vi "User.vi"() -> ()   [LabVIEW 2023]
uses:
  Tab_typeDef_user.ctl
  Global 1.vi
  <vilib>/Utility/file.llb/Read Delimited Spreadsheet (string).vi
  <vilib>/Utility/file.llb/Write Delimited Spreadsheet (string).vi
panel:
  in  "Tab Control":T1(tab)=enum."Registration"
  out "String":string
  in  "register_btn":bool
  in  "login_btn":bool
  in  "password_login":string
  in  "username_login":string
  in  "home_btn":bool
  in  "Location_of_locker":u16(ring) items=["Choose location", "ul. Arkuszowa 109, 01-934 Warszawa", "ul. Polczynska 104, 01-302 Warszawa"]
  in  "Send_Button":bool
  in  "Receive_Button":bool caption="Send_Button"
  in  "back_to_login_btn":bool
  out "rgstr_status":string
  in  "email_address_rgstr":string
  in  "last_name_rgstr":string
  in  "first_name_rgstr":string
  in  "register_btn_rgstr":bool
  in  "password_rgstr":string
  in  "username_rgstr":string
  in  "pickup_btn_rcv":bool
  in  "menu_btn_rcv":bool
  in  "pickup_code_rcv_1":string
  in  "phone_receiver_rcv_1":string
  in  "radio_btn_sizes_of_parcel 2":T2(radio)
  in  "Location_of_locker_rcp":u16(ring) items=["Choose location", "ul. Arkuszowa 109, 01-934 Warszawa", "ul. Polczynska 104, 01-302 Warszawa"]
  in  "Location_of_locker_sender_send":u16(ring) items=["Choose location", "ul. Arkuszowa 109, 01-934 Warszawa", "ul. Polczynska 104, 01-302 Warszawa"]
  in  "recipient_phone_send":string
  in  "sender_phone_number_send":string
  in  "next_btn_send":bool
  in  "back_btn_send":bool
  # "User:"
  # "Login"
  # "Thanks for choosing\nParcelFast"
  # "Username:"
  # "Use our system in two steps:"
  # "Password:"
  # "1. Select your current location: B"
  # "2. Do you want to send or receive a package?"
  # "or Register"
  # "Registration"
  # "First Name:"
  # "Last Name:"
  # "Email Address:"
  # "Username:"
  # "Password:"
  # "Fill in the required gaps below:"
  # "Phone number:"
  # "Pickup-code:"
  # "Confirm your details:"
  # "You:"
  # "Phone number:"
  # "Destination:"
  # "Recipient:"
  # "Phone number:"
  # "Destination:"
  # "Min size"
  # "Medium size"
  # "Big size"
  # "Price 15,00 zl"
  # "Price 18,99 zl"
  # "Price 18,99 zl"
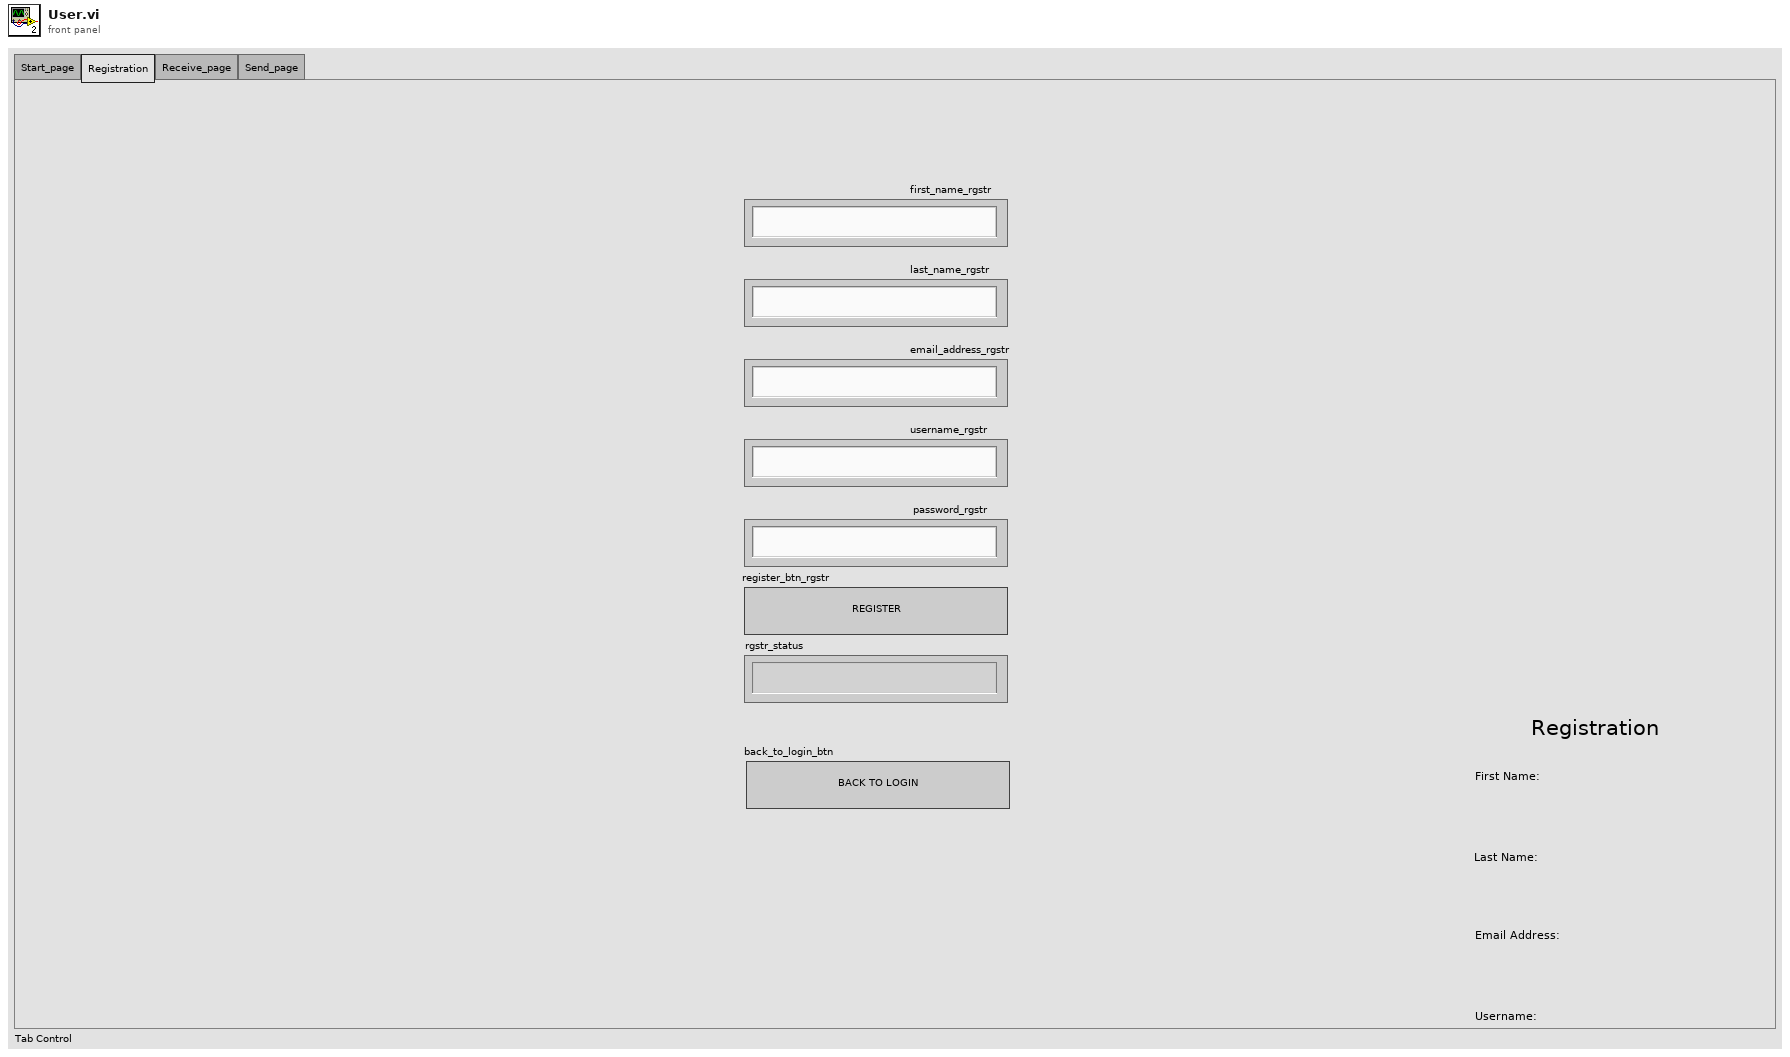
[diagram p1: front panel]
types:
  T1 = enum32{"Start_page", "Registration", "Receive_page", "Send_page"}
  T2 = enum32{"Radio Selection 1", "Radio Selection 2", "Radio Selection 3"}
  T3 = typedef "Tab_typeDef_user.ctl" = enum32{"Start_page", "Registration", "Receive_page", "Send_page"}
  T4 = cluster{bool, "tab_control_user ":T3, "phone_receiver":string, "pickup_code_receiver":string, "time_start_rcv":timestamp, "time_end_rcv":timestamp, "time_start_send":timestamp, "time_end_send":timestamp, "your_phone_receiver":string, "recipients_phone_receiver":string, "radio_btn_size":i32, "Probe":i32}
  T5 = enum16{"open", "replace", "create", "open or create", "replace or create", "replace or create with confirmation"}
  T6 = typedef "Tab_typeDef_lock_state.ctl" = u16
  T7 = cluster{"id_locker":i32, "lock_state":T6, "array_of_boxes_of_locker":cluster{"parcel_end_time":timestamp, "parcel_placement_time":timestamp, "box_filling":dbl, "adres_to send_parcel":i32}[][], "num_parcel":dbl[]}[]
  T8 = cluster{"id_locker":i32, "lock_state":T6, "array_of_boxes_of_locker":cluster{"parcel_end_time":timestamp, "parcel_placement_time":timestamp, "box_filling":dbl, "adres_to send_parcel":i32}[][], "num_parcel":dbl[]}
  T9 = cluster{"parcel_end_time":timestamp, "parcel_placement_time":timestamp, "box_filling":dbl, "adres_to send_parcel":i32}[][]
  T10 = cluster{"parcel_end_time":timestamp, "parcel_placement_time":timestamp, "box_filling":dbl, "adres_to send_parcel":i32}[]
  T11 = cluster{"parcel_end_time":timestamp, "parcel_placement_time":timestamp, "box_filling":dbl, "adres_to send_parcel":i32}
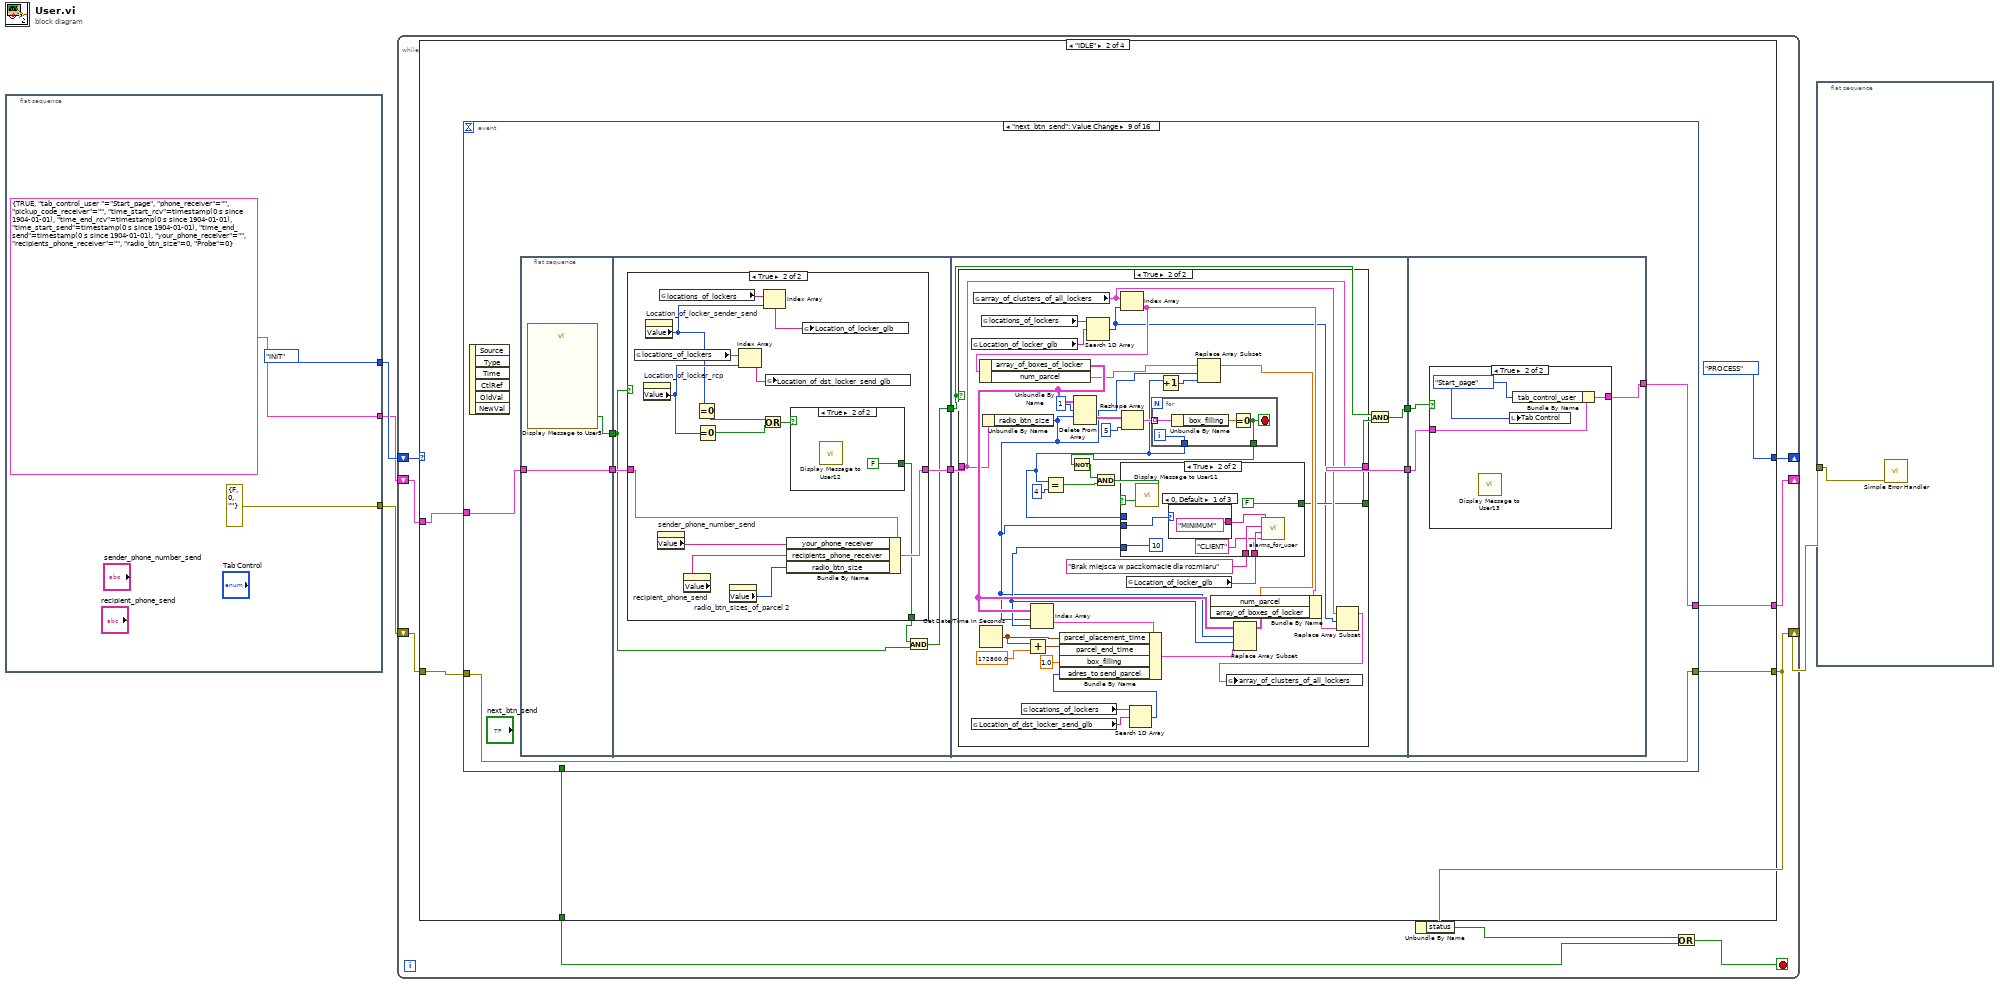
[diagram p0: block diagram]
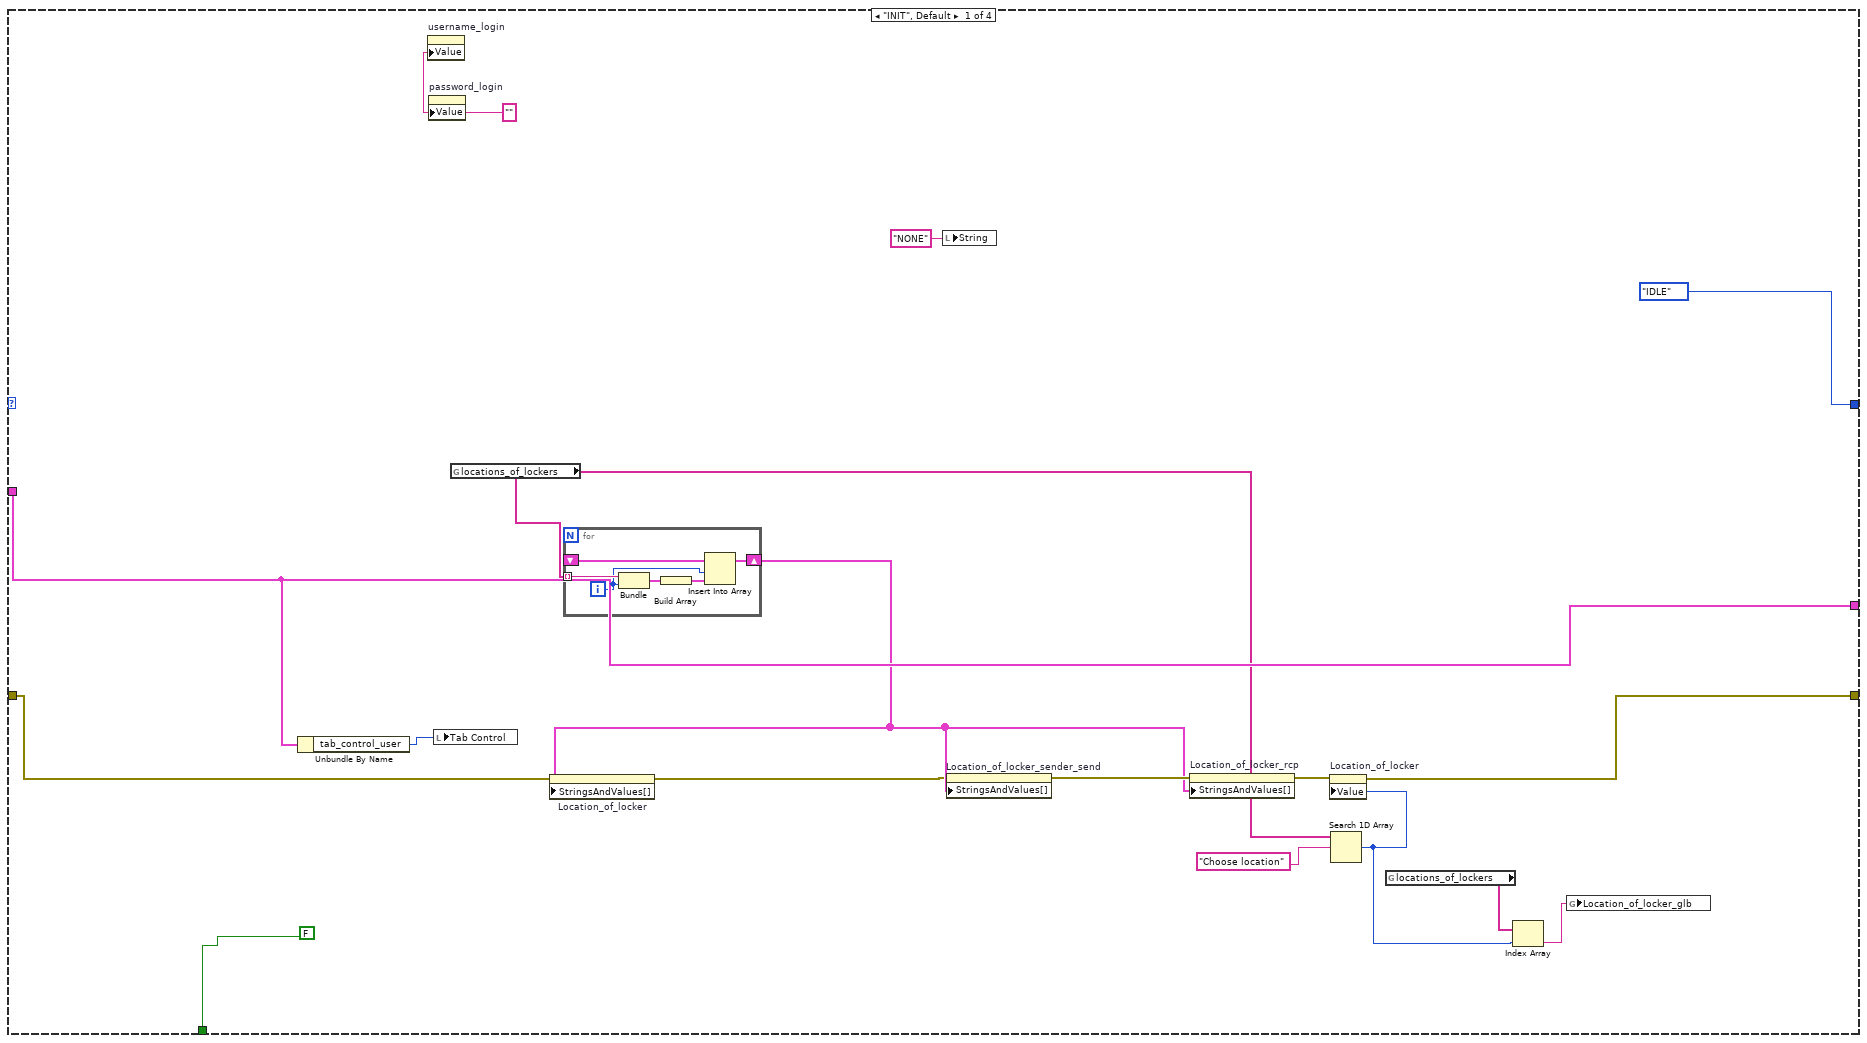
[diagram p2: hidden frame]
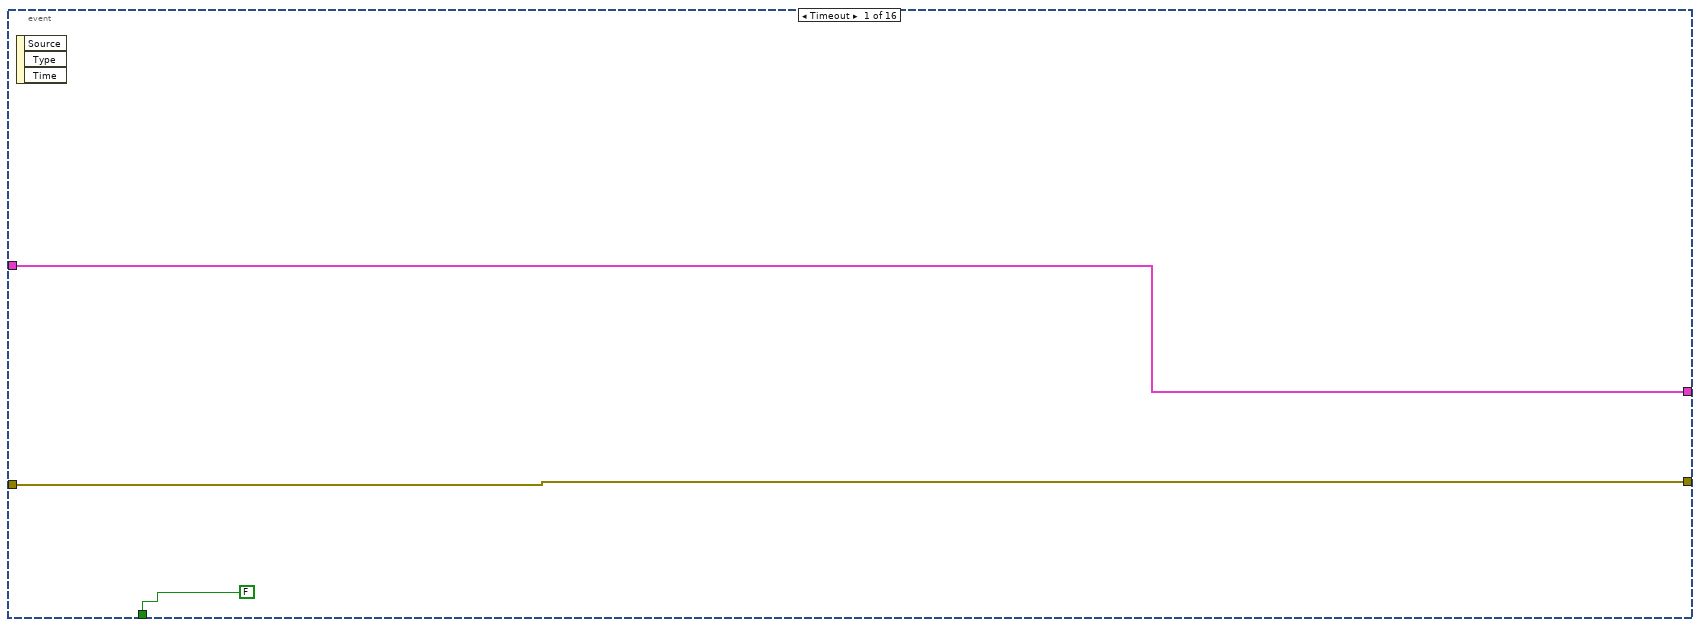
[diagram p3: hidden frame]
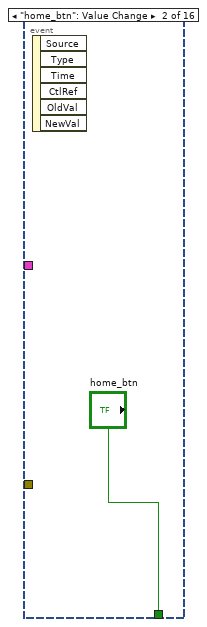
[diagram p4: hidden frame]
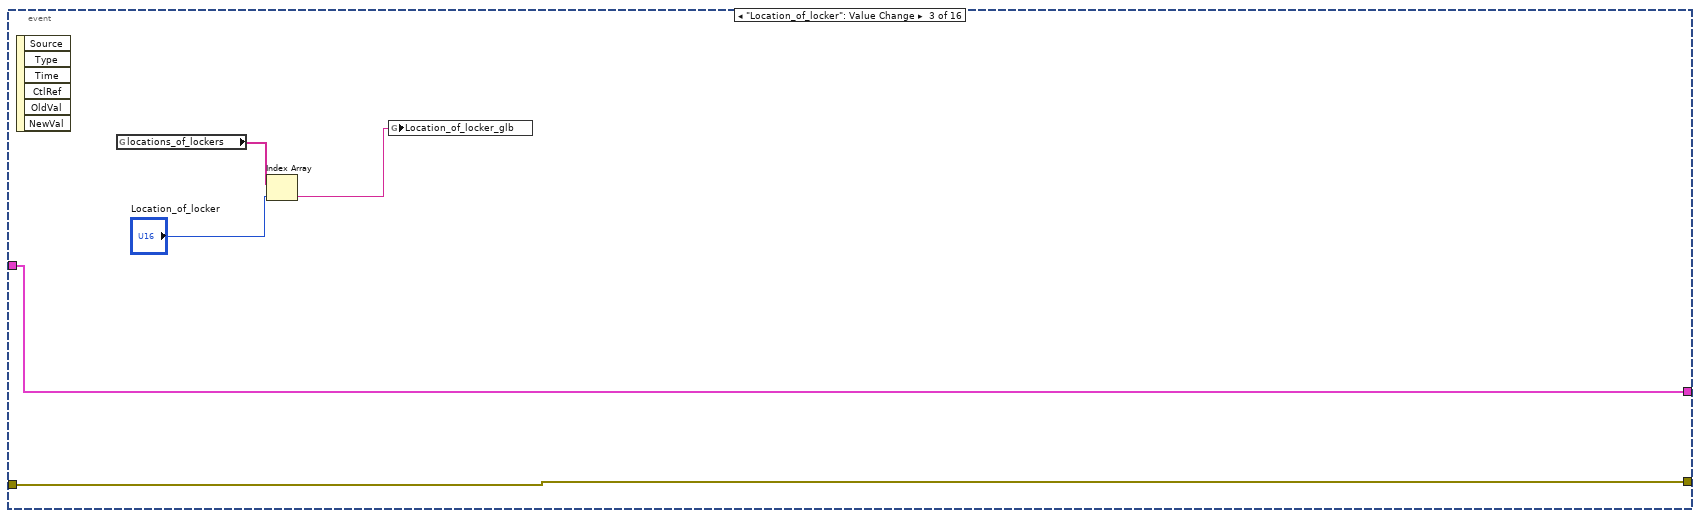
[diagram p5: hidden frame]
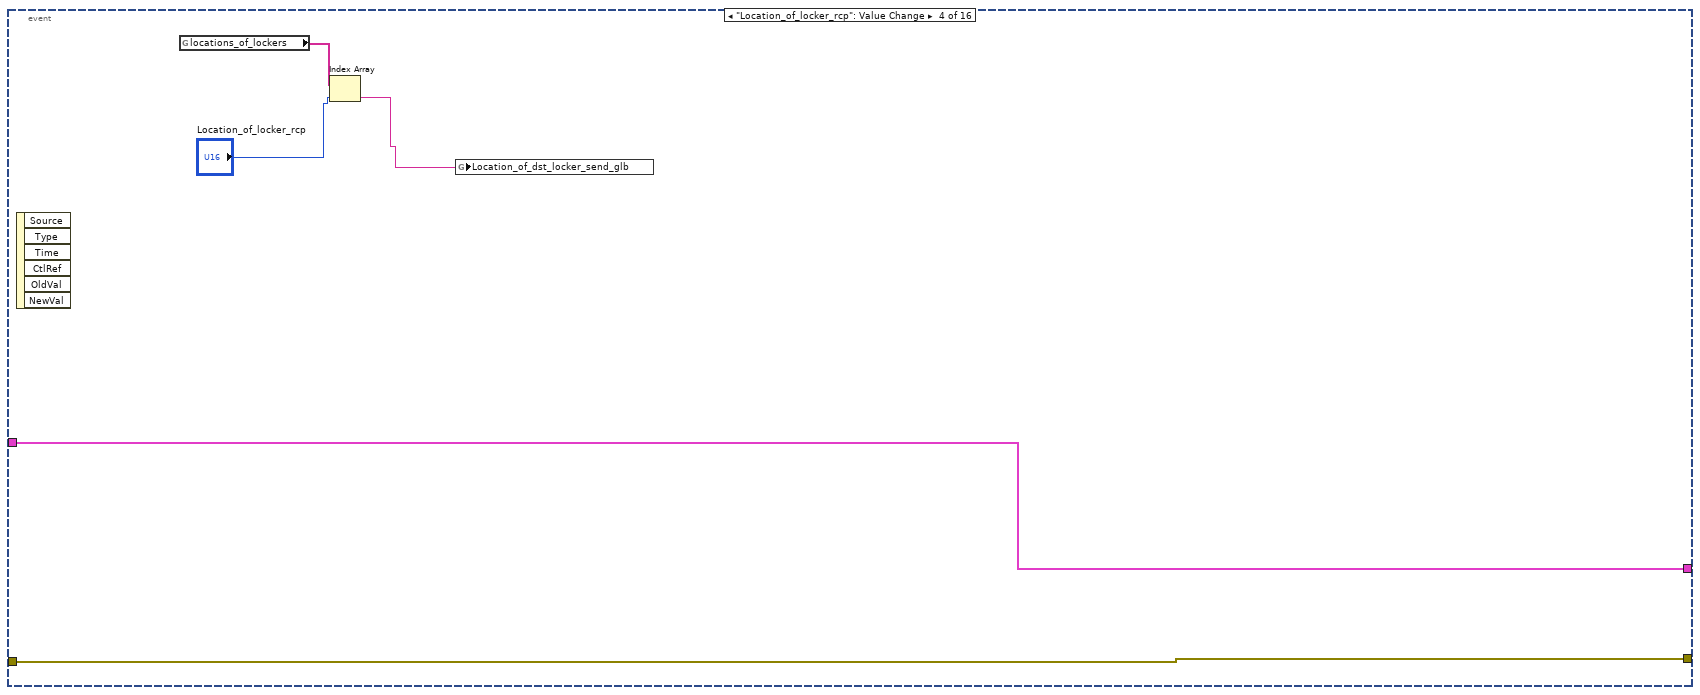
[diagram p6: hidden frame]
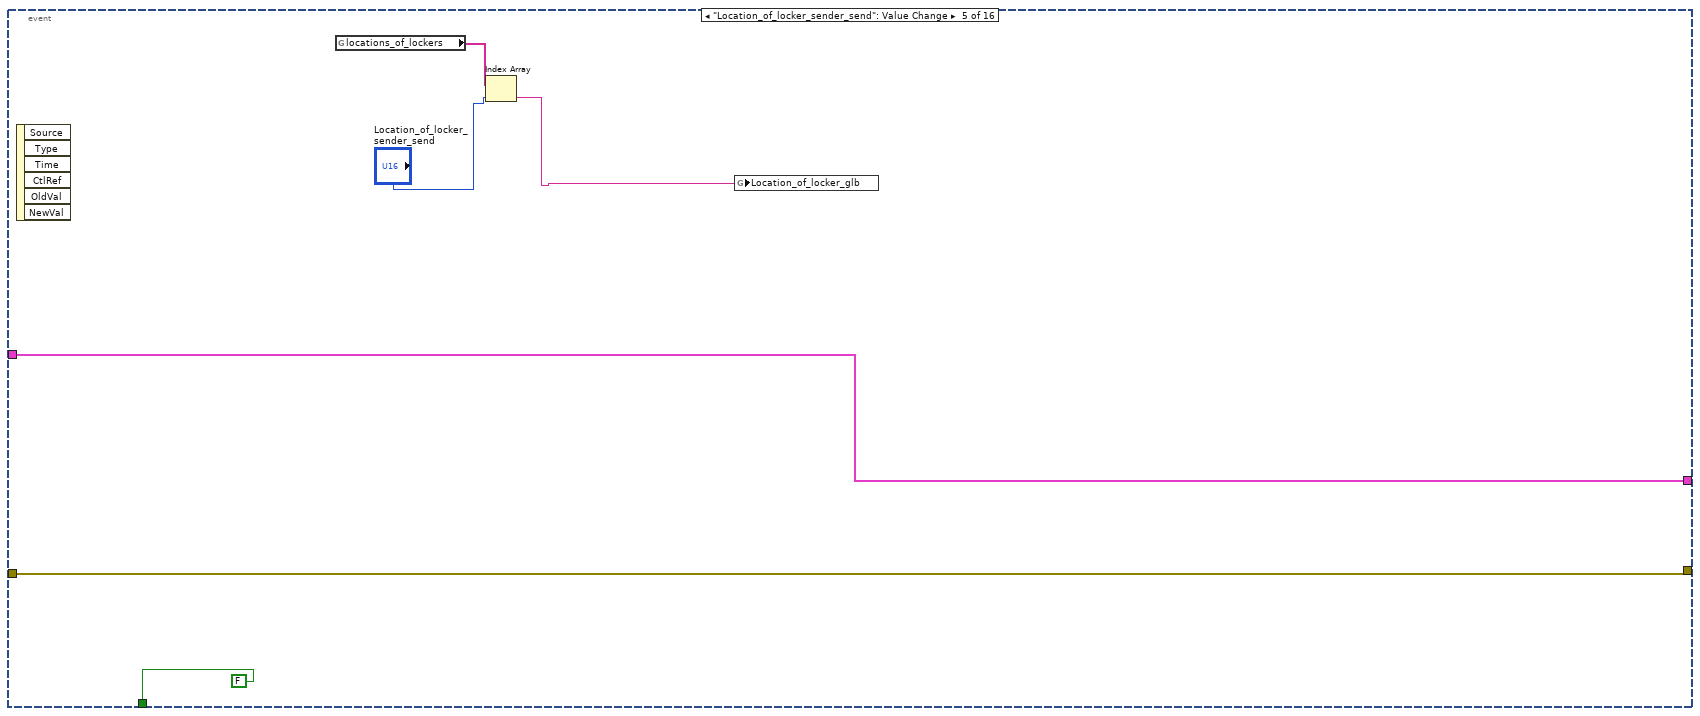
[diagram p7: hidden frame]
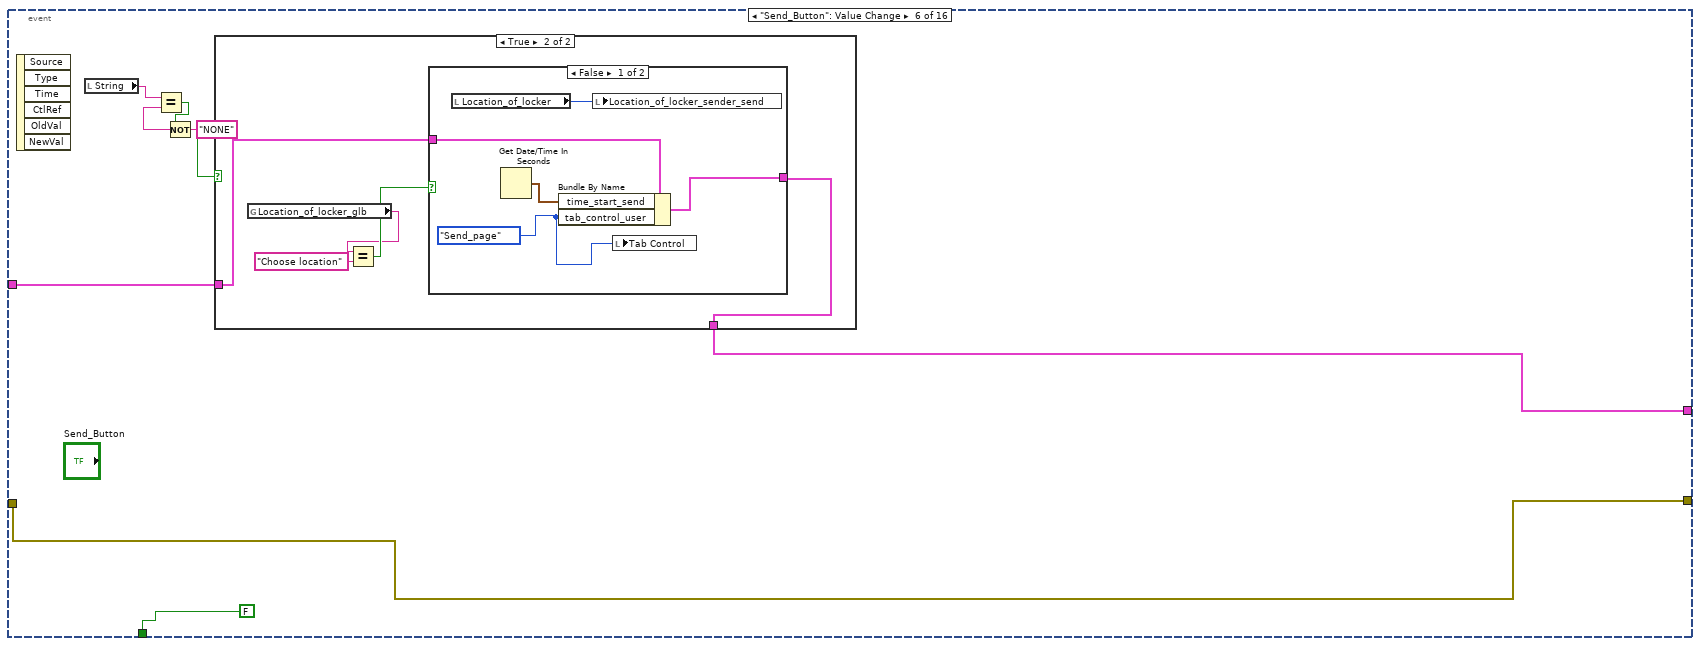
[diagram p8: hidden frame]
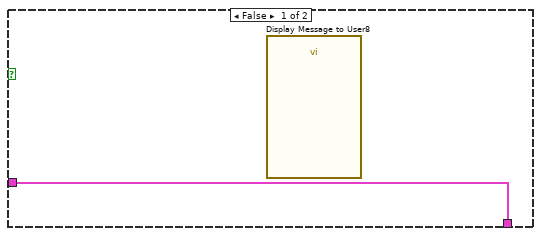
[diagram p9: hidden frame]
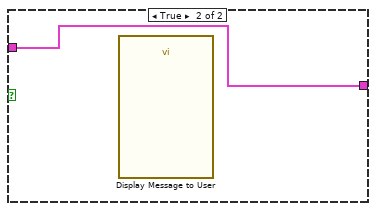
[diagram p10: hidden frame]
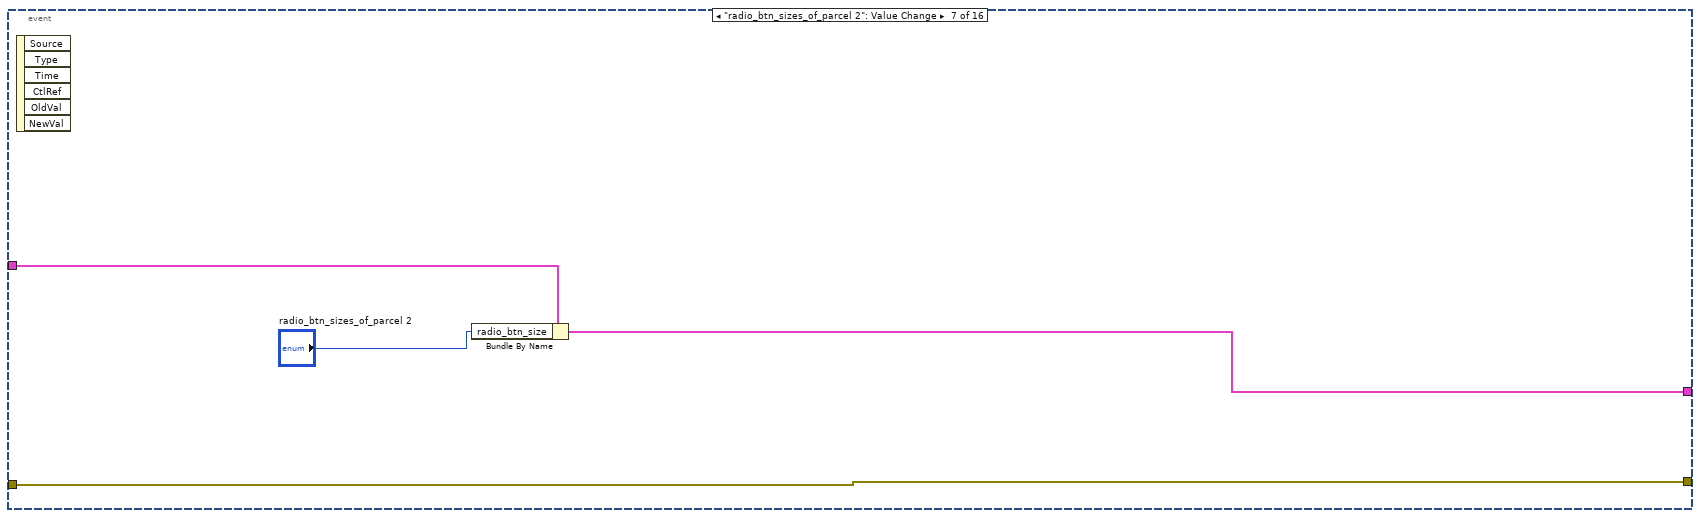
[diagram p11: hidden frame]
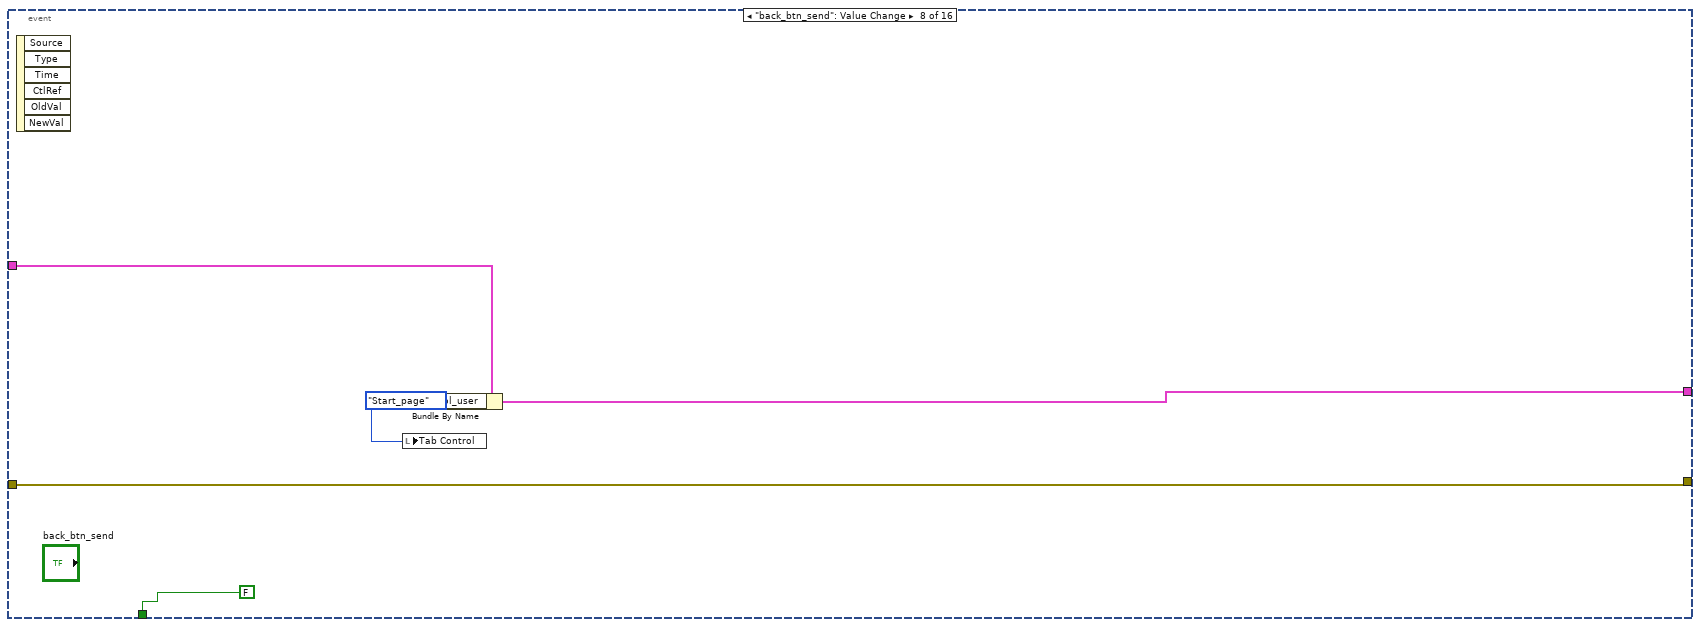
[diagram p12: hidden frame]
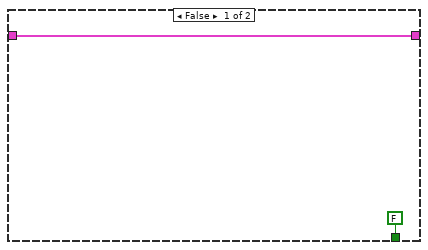
[diagram p13: hidden frame]
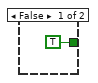
[diagram p14: hidden frame]
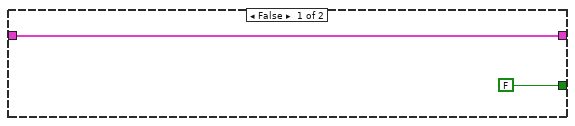
[diagram p15: hidden frame]
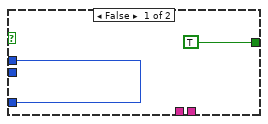
[diagram p16: hidden frame]
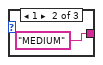
[diagram p17: hidden frame]
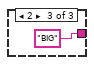
[diagram p18: hidden frame]
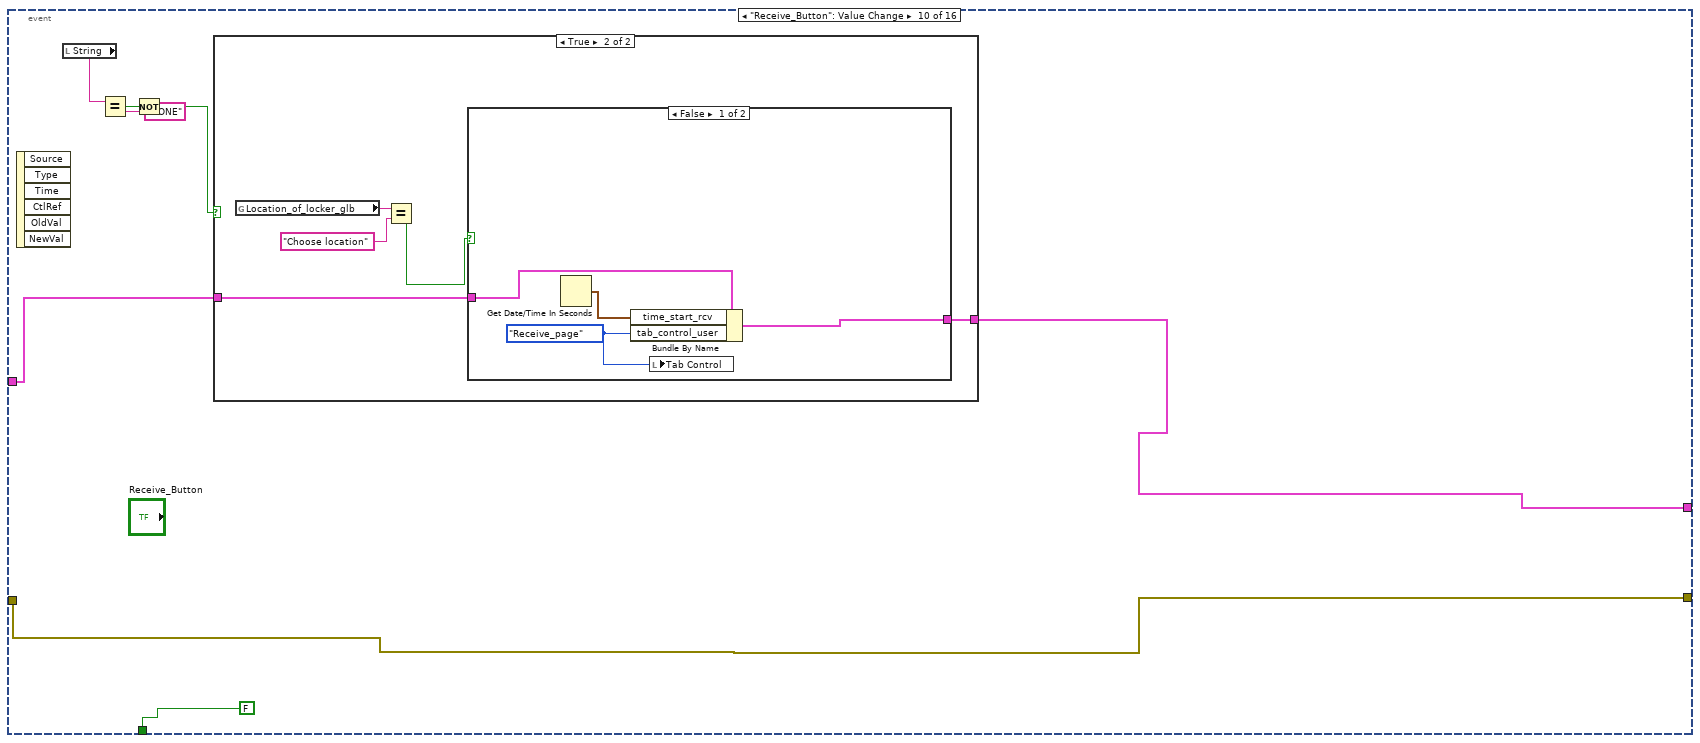
[diagram p20: hidden frame]
diagram:
  n1 = flat-sequence {
    tunnel: [errorcluster {"status"=FALSE, "code"=0, "source"=""} ("error constant")] -> w3
    tunnel: [enum16{"INIT", "IDLE", "PROCESS", "EXIT"}."INIT"] -> w4
    tunnel: [T4 {TRUE, "tab_control_user "=enum."Start_page", "phone_receiver"="", "pickup_code_receiver"="", "time_start_rcv"=timestamp(0 s since 1904-01-01), "time_end_rcv"=timestamp(0 s since 1904-01-01), "time_start_send"=timestamp(0 s since 1904-01-01), "time_end_send"=timestamp(0 s since 1904-01-01), "your_phone_receiver"="", "recipients_phone_receiver"="", "radio_btn_size"=0, "Probe"=0}] -> w1
    frame #0 {
    }
  }
  n2 = while {
    shift-right: [w15] -> _
    shift-left: w4 -> [w16]
    shift-right: [w14] -> _
    shift-left: w1 -> [w9]
    shift-right: [w11] -> w2
    shift-left: w3 -> [w8]
    stop <- w10 stop-if-true
    n3 = case shown="\"IDLE\"" w16 {
      tunnel: [enum16{"INIT", "IDLE", "PROCESS", "EXIT"}."IDLE" enum16{"INIT", "IDLE", "PROCESS", "EXIT"}."PROCESS" enum16{"INIT", "IDLE", "PROCESS", "EXIT"}."IDLE" enum16{"INIT", "IDLE", "PROCESS", "EXIT"}."EXIT"] -> w15
      tunnel: [FALSE ("stop") w44 FALSE ("stop") TRUE ("stop")] -> w12
      tunnel: [w31 w43 w395 w399] -> w14
      tunnel: [w21 w41 w394 w398] -> w11
      tunnel: w9 -> [w31 w42 w395 w399]
      tunnel: w8 -> [w29 w40 w394 w398]
      frame "INIT", Default {
        w17 = "" ("password_login")
        n4 = Unbundle By Name(w31) -> ("tab_control_user"=w30:T3)
        n5 = property on="username_login" class="Str"("Value"=w17) -> ()  [unwired: 2 in, 2 out]
        n6 = property on="password_login" class="Str"("Value"=w17) -> ()  [unwired: 2 in, 2 out]
        n7 = local write "Tab Control"(w30) -> ()
        n8 = global read "Global 1.vi" "locations_of_lockers"() -> (w23:string[])
        n9 = for {
          tunnel: w23 -> [w39] mode=indexing
          shift-right: [w36] -> w25
          shift-left: _ -> [w37]
          i -> [w34]
          n10 = Bundle("String"=w39, w34) -> (w38:cluster{"String":string, i32})  [unwired: 1 in]
          n11 = Build Array(w38) -> (w35:cluster{"String":string, i32}[])
          n12 = Insert Into Array(array=w37, index=w34, new element=w35) -> (w36:cluster{"String":string, i32}[])
        }
        n13 = property on="Location_of_locker" class="Ring (strict)"(error in=w29, "StringsAndValues[]"=w25) -> (error out=w22:errorcluster)  [unwired: 1 in, 1 out]
        n14 = local write "String"("NONE" ("String")) -> ()
        n15 = property on="Location_of_locker_sender_send" class="Ring (strict)"(error in=w22, "StringsAndValues[]"=w25) -> (error out=w27:errorcluster)  [unwired: 1 in, 1 out]
        n16 = property on="Location_of_locker_rcp" class="Ring (strict)"(error in=w27, "StringsAndValues[]"=w25) -> (error out=w26:errorcluster)  [unwired: 1 in, 1 out]
        n17 = Search 1D Array(1D array=w23, element="Choose location" ("new element/subarray")) -> (index of element=w18:i32)  [unwired: 1 in]
        n18 = property on="Location_of_locker" class="Ring (strict)"(error in=w26, "Value"=w18) -> (error out=w21:errorcluster)  [unwired: 1 in, 1 out]
        n19 = global read "Global 1.vi" "locations_of_lockers"() -> (w20:string[])
        n20 = Index Array(array=w20, index=w18) -> (element=w19:string)
        n21 = global write "Global 1.vi" "Location_of_locker_glb"(w19) -> ()
      }
      frame "IDLE" {
        n22 = event shown="[8] \"next_btn_send\": Value Change" {
          selector: _ -> [_ _ _ _ _ _ _ _ _ _ _ _ _ _ _ _]
          dyn-events: _ -> [_ _ _ _ _ _ _ _ _ _ _ _ _ _ _ _]
          timeout: _ -> [_ _ _ _ _ _ _ _ _ _ _ _ _ _ _ _]
          tunnel: [FALSE ("stop") "home_btn" _ _ FALSE ("home_btn") FALSE ("home_btn") _ FALSE ("home_btn") _ FALSE ("home_btn") FALSE ("home_btn") _ _ _ _ _] -> w44
          tunnel: [w47 _ w54 w58 w63 w71 w87 w91 w99 w203 w217 w225 w228 w306 _ w391] -> w43
          tunnel: w42 -> [w47 _ w54 w58 w63 w72 w89 w92 w102 w204 w218 w223 w231 w308 _ w393]
          tunnel: [w46 _ w53 w59 w64 w70 w86 w93 w103 w202 _ _ w226 w299 _ w388] -> w41
          tunnel: w40 -> [w46 _ w53 w59 w64 w70 w86 w93 w103 w202 _ _ w226 w300 _ w390]
          event Timeout {
            n23 = event-data() -> ()  [unwired: 1 in, 3 out]
          }
          event "home_btn": Value Change {
            n24 = event-data() -> ()  [unwired: 1 in, 6 out]
          }
          event "Location_of_locker": Value Change {
            n25 = event-data() -> ()  [unwired: 1 in, 6 out]
            n26 = global read "Global 1.vi" "locations_of_lockers"() -> (w51:string[])
            n27 = Index Array(array=w51, index="Location_of_locker") -> (element=w50:string)
            n28 = global write "Global 1.vi" "Location_of_locker_glb"(w50) -> ()
          }
          event "Location_of_locker_rcp": Value Change {
            n29 = event-data() -> ()  [unwired: 1 in, 6 out]
            n30 = global read "Global 1.vi" "locations_of_lockers"() -> (w57:string[])
            n31 = Index Array(array=w57, index="Location_of_locker_rcp") -> (element=w55:string)
            n32 = global write "Global 1.vi" "Location_of_dst_locker_send_glb"(w55) -> ()
          }
          event "Location_of_locker_sender_send": Value Change {
            n33 = event-data() -> ()  [unwired: 1 in, 6 out]
            n34 = global read "Global 1.vi" "locations_of_lockers"() -> (w62:string[])
            n35 = Index Array(array=w62, index="Location_of_locker_sender_send") -> (element=w60:string)
            n36 = global write "Global 1.vi" "Location_of_locker_glb"(w60) -> ()
          }
          event "Send_Button": Value Change {
            n37 = event-data() -> ()  [unwired: 1 in, 6 out]
            n38 = local read "String"() -> (w69:string)
            n39 = Equal?(x=w69, y="NONE") -> (x = y?=w67:bool)
            n40 = Not(x=w67) -> (.not. x?=w66:bool)
            n41 = case shown="True" w66 {
              tunnel: w72 -> [w74 w77]
              tunnel: [w74 w76] -> w71
              frame False {
                n42 = call "Display Message to User8"() -> ()  [unwired: 10 in, 2 out]
              }
              frame True {
                n43 = global read "Global 1.vi" "Location_of_locker_glb"() -> (w75:string)
                n44 = Equal?(x=w75, y="Choose location") -> (x = y?=w78:bool)
                n45 = case shown="False" w78 {
                  tunnel: w77 -> [w84 w85]
                  tunnel: [w83 w85] -> w76
                  frame False {
                    w81 = Tab_typeDef_user."Send_page" ("tab_control_user")
                    n46 = local read "Location_of_locker"() -> (w80:u16)
                    n47 = Get Date/Time In Seconds() -> (seconds since 1Jan1904=w82:timestamp)
                    n48 = Bundle By Name(cluster=w84, "time_start_send"=w82, "tab_control_user"=w81) -> (w83:T4)
                    n49 = local write "Location_of_locker_sender_send"(w80) -> ()
                    n50 = local write "Tab Control"(w81) -> ()
                  }
                  frame True {
                    n51 = call "Display Message to User"() -> ()  [unwired: 10 in, 2 out]
                  }
                }
              }
            }
          }
          event "radio_btn_sizes_of_parcel 2": Value Change {
            n52 = event-data() -> ()  [unwired: 1 in, 6 out]
            n53 = Bundle By Name(cluster=w89, "radio_btn_size"="radio_btn_sizes_of_parcel 2") -> (w87:T4)
          }
          event "back_btn_send": Value Change {
            w90 = Tab_typeDef_user."Start_page" ("tab_control_user")
            n54 = event-data() -> ()  [unwired: 1 in, 6 out]
            n55 = Bundle By Name(cluster=w92, "tab_control_user"=w90) -> (w91:T4)
            n56 = local write "Tab Control"(w90) -> ()
          }
          event "next_btn_send": Value Change {
            n57 = event-data() -> ()  [unwired: 1 in, 6 out]
            n58 = flat-sequence {
              tunnel: w102 -> [w105]
              tunnel: [w105] -> w101
              tunnel: [w104] -> w100
              tunnel: w101 -> [w110]
              tunnel: [w109] -> w98
              tunnel: [w106] -> w96
              tunnel: w100 -> [w107]
              tunnel: w98 -> [w134]
              tunnel: [w133] -> w97
              tunnel: w96 -> [w132]
              tunnel: [w131] -> w95
              tunnel: [w191] -> w99
              tunnel: w97 -> [w192]
              tunnel: w95 -> [w190]
              frame #0 {
                n59 = call "Display Message to User5"() -> ("OK"=w104:bool)  [unwired: 10 in, 1 out]
              }
              frame #1 {
                n60 = case shown="True" w107 {
                  tunnel: w110 -> [w112 w127]
                  tunnel: [w112 w124] -> w109
                  tunnel: [FALSE w113] -> w108
                  frame False {
                  }
                  frame True {
                    n61 = global read "Global 1.vi" "locations_of_lockers"() -> (w121:string[])
                    n62 = property on="Location_of_locker_rcp" class="Ring (strict)"() -> ("Value"=w118:u16)  [unwired: 2 in, 2 out]
                    n63 = property on="Location_of_locker_sender_send" class="Ring (strict)"() -> ("Value"=w116:u16)  [unwired: 2 in, 2 out]
                    n64 = property on="sender_phone_number_send" class="Str"() -> ("Value"=w126:string)  [unwired: 2 in, 2 out]
                    n65 = global read "Global 1.vi" "locations_of_lockers"() -> (w123:string[])
                    n66 = property on="recipient_phone_send" class="Str"() -> ("Value"=w125:string)  [unwired: 2 in, 2 out]
                    n67 = Equal To 0?(x=w116) -> (x = 0?=w115:bool)
                    n68 = Equal To 0?(x=w118) -> (x = 0?=w114:bool)
                    n69 = property on="radio_btn_sizes_of_parcel 2" class="RadioBtnsControl (strict)"() -> ("Value"=w119:T2)  [unwired: 2 in, 2 out]
                    n70 = Index Array(array=w121, index=w118) -> (element=w120:string)
                    n71 = Or(x=w115, y=w114) -> (x .or. y?=w117:bool)
                    n72 = Index Array(array=w123, index=w116) -> (element=w122:string)
                    n73 = global write "Global 1.vi" "Location_of_dst_locker_send_glb"(w120) -> ()
                    n74 = Bundle By Name(cluster=w127, "your_phone_receiver"=w126, "recipients_phone_receiver"=w125, "radio_btn_size"=w119) -> (w124:T4)
                    n75 = case shown="True" w117 {
                      tunnel: [TRUE FALSE] -> w113
                      frame False {
                      }
                      frame True {
                        n76 = call "Display Message to User12"() -> ()  [unwired: 10 in, 2 out]
                      }
                    }
                    n77 = global write "Global 1.vi" "Location_of_locker_glb"(w122) -> ()
                  }
                }
                n78 = And(x=w108, y=w107) -> (x .and. y?=w106:bool)
              }
              frame #2 {
                n79 = case shown="True" w132 {
                  tunnel: w134 -> [w136 w146]
                  tunnel: [w136 w146] -> w133
                  tunnel: [FALSE w147] -> w130
                  frame False {
                  }
                  frame True {
                    n80 = global read "Global 1.vi" "Location_of_locker_glb"() -> (w172:string)
                    n81 = global read "Global 1.vi" "Location_of_dst_locker_send_glb"() -> (w141:string)
                    n82 = global read "Global 1.vi" "array_of_clusters_of_all_lockers"() -> (w158:T7)
                    n83 = Get Date/Time In Seconds() -> (seconds since 1Jan1904=w164:timestamp)
                    n84 = global read "Global 1.vi" "locations_of_lockers"() -> (w173:string[])
                    n85 = Unbundle By Name(w146) -> ("radio_btn_size"=w139:i32)
                    n86 = global read "Global 1.vi" "locations_of_lockers"() -> (w142:string[])
                    n87 = Add(x=w164, y=172800.0) -> (x+y=w165:timestamp)
                    n88 = Search 1D Array(1D array=w173, element=w172) -> (index of element=w143:i32)  [unwired: 1 in]
                    n89 = Index Array(array=w158, index=w143) -> (element=w160:T8)
                    n90 = Unbundle By Name(w160) -> ("array_of_boxes_of_locker"=w162:T9, "num_parcel"=w155:dbl[])
                    n91 = Delete From Array(array=w162, length=1, index (row)=w139) -> (deleted portion=w170:T9)  [unwired: 1 in, 1 out]
                    n92 = Reshape Array(w170, 5 ("dimension size")) -> (w168:T10)
                    n93 = global read "Global 1.vi" "Location_of_locker_glb"() -> (w137:string)
                    n94 = Search 1D Array(1D array=w142, element=w141) -> (index of element=w140:i32)  [unwired: 1 in]
                    n95 = for {
                      tunnel: w168 -> [w189] mode=indexing
                      tunnel: [w187] -> w145
                      tunnel: [w186] -> w150
                      i -> [w187]
                      stop <- w186 stop-if-true
                      n96 = Unbundle By Name(w189) -> ("box_filling"=w188:dbl)
                      n97 = Equal To 0?(x=w188) -> (x = 0?=w186:bool)
                    }
                    n98 = Equal?(x=w145, y=4) -> (x = y?=w152:bool)
                    n99 = Not(x=w150) -> (.not. x?=w149:bool)
                    n100 = And(x=w149, y=w152) -> (x .and. y?=w151:bool)
                    n101 = case shown="True" w151 {
                      tunnel: w145 -> [w175 _]
                      tunnel: [w175 10] -> w148
                      tunnel: [TRUE FALSE] -> w147
                      tunnel: w139 -> [_ w180]
                      tunnel: "Brak miejsca w paczkomacie dla rozmiaru" -> [_ w178]
                      tunnel: w137 -> [_ w179]
                      frame False {
                      }
                      frame True {
                        n102 = call "Display Message to User11"() -> ()  [unwired: 10 in, 2 out]
                        n103 = case shown="0, Default" w180 {
                          tunnel: ["MINIMUM" "MEDIUM" "BIG"] -> w177
                          frame 0, Default {
                          }
                          frame 1 {
                          }
                          frame 2 {
                          }
                        }
                        n104 = call "alarms_for_user.vi"("name_user_option"="CLIENT", "adres"=w179, "texxt_alarm"=w178, "size_name"=w177) -> ()  [unwired: 8 in]
                      }
                    }
                    n105 = Index Array(array=w162, index (row)=w139, index (col)=w148) -> (element=w167:T11)
                    n106 = Bundle By Name(cluster=w167, "parcel_placement_time"=w164, "parcel_end_time"=w165, "box_filling"=1.0, "adres_to send_parcel"=w140) -> (w161:T11)
                    n107 = Increment(x=w145) -> (x+1=w144:i32)
                    n108 = Replace Array Subset(array=w155, new element=w144, index=w139) -> (w154:dbl[])
                    n109 = Replace Array Subset(array=w162, new element=w161, index (row)=w139, index (col)=w148) -> (w159:T9)
                    n110 = Bundle By Name(cluster=w160, "num_parcel"=w154, "array_of_boxes_of_locker"=w159) -> (w157:T8)
                    n111 = Replace Array Subset(array=w158, new element=w157, index=w143) -> (w156:T7)
                    n112 = global write "Global 1.vi" "array_of_clusters_of_all_lockers"(w156) -> ()
                  }
                }
                n113 = And(x=w132, y=w130) -> (x .and. y?=w131:bool)
              }
              frame #3 {
                n114 = case shown="True" w190 {
                  tunnel: w192 -> [w193 w196]
                  tunnel: [w193 w194] -> w191
                  frame False {
                  }
                  frame True {
                    w195 = Tab_typeDef_user."Start_page" ("tab_control_user")
                    n115 = call "Display Message to User13"() -> ()  [unwired: 10 in, 2 out]
                    n116 = local write "Tab Control"(w195) -> ()
                    n117 = Bundle By Name(cluster=w196, "tab_control_user"=w195) -> (w194:T4)
                  }
                }
              }
            }
          }
          event "Receive_Button": Value Change {
            n118 = event-data() -> ()  [unwired: 1 in, 6 out]
            n119 = local read "String"() -> (w200:string)
            n120 = Equal?(x=w200, y="NONE") -> (x = y?=w198:bool)
            n121 = Not(x=w198) -> (.not. x?=w197:bool)
            n122 = case shown="True" w197 {
              tunnel: w204 -> [w205 w207]
              tunnel: [w205 w206] -> w203
              frame False {
                n123 = call "Display Message to User9"() -> ()  [unwired: 10 in, 2 out]
              }
              frame True {
                n124 = global read "Global 1.vi" "Location_of_locker_glb"() -> (w209:string)
                n125 = Equal?(x=w209, y="Choose location") -> (x = y?=w208:bool)
                n126 = case shown="False" w208 {
                  tunnel: w207 -> [w214 w215]
                  tunnel: [w213 w215] -> w206
                  frame False {
                    w212 = Tab_typeDef_user."Receive_page" ("tab_control_user")
                    n127 = Get Date/Time In Seconds() -> (seconds since 1Jan1904=w211:timestamp)
                    n128 = Bundle By Name(cluster=w214, "time_start_rcv"=w211, "tab_control_user"=w212) -> (w213:T4)
                    n129 = local write "Tab Control"(w212) -> ()
                  }
                  frame True {
                    n130 = call "Display Message to User2"() -> ()  [unwired: 10 in, 2 out]
                  }
                }
              }
            }
          }
          event "menu_btn_rcv": Value Change {
            w216 = Tab_typeDef_user."Start_page" ("tab_control_user")
            n131 = event-data() -> ()  [unwired: 1 in, 6 out]
            n132 = Bundle By Name(cluster=w218, "tab_control_user"=w216) -> (w217:T4)
            n133 = local write "Tab Control"(w216) -> ()
          }
          event "pickup_btn_rcv": Value Change {
            w224 = Tab_typeDef_user."Start_page" ("tab_control_user")
            n134 = event-data() -> ()  [unwired: 1 in, 6 out]
            n135 = Bundle By Name(cluster=w223, "phone_receiver"="phone_receiver_rcv_1", "pickup_code_receiver"="pickup_code_rcv_1") -> (w220:T4)
            n136 = Bundle By Name(cluster=w220, "tab_control_user"=w224) -> (w225:T4)
            n137 = local write "Tab Control"(w224) -> ()
          }
          event "login_btn": Value Change {
            n138 = event-data() -> ()  [unwired: 1 in, 6 out]
            n139 = call <vilib>:"Application Directory.vi"() -> ("Application Directory"=w237:path)
            n140 = Path To String(path=w237) -> (string=w236:string)
            n141 = Concatenate Strings(w236, "\\databases\\") -> (w234:string)
            n142 = String To Path(string=w234) -> (path=w233:path)
            n143 = Build Path(base path=w233, name or relative path="Clients_database.csv") -> (appended path=w232:path)
            n144 = call-poly <vilib>:"Read Delimited Spreadsheet.vi"("file path (dialog if empty)"=w232, "delimiter (\\t)"="," ("delimiter (\\t)")) -> ("all rows"=w239:string[][])  [unwired: 8 in, 5 out]
            n145 = for {
              tunnel: w239 -> [w297] mode=indexing
              tunnel: "username_login" -> [w296]
              tunnel: "password_login" -> [w295]
              tunnel: [w292] -> w227
              stop <- w292 stop-if-true
              n146 = Index Array(array=w297) -> (element #4=w290:string, element #5=w291:string)  [unwired: 5 in, 3 out]
              n147 = Equal?(x=w290, y=w296) -> (x = y?=w294:bool)
              n148 = Equal?(x=w291, y=w295) -> (x = y?=w293:bool)
              n149 = And(x=w294, y=w293) -> (x .and. y?=w292:bool)
            }
            n150 = case shown="False" w227 {
              tunnel: w231 -> [w244 w289]
              tunnel: [w245 w288] -> w228
              tunnel: "username_login" -> [w252 w286]
              tunnel: "password_login" -> [w249 _]
              frame False {
                n151 = Unbundle By Name(w244) -> ("Probe"=w241:i32)
                n152 = Equal?(x=w241, y=3) -> (x = y?=w242:bool)
                n153 = case shown="True" w242 {
                  tunnel: [w255 w258] -> w245
                  tunnel: w244 -> [w256 w259]
                  tunnel: w241 -> [w253 _]
                  frame False {
                    n154 = Increment(x=w253) -> (x+1=w254:i32)
                    n155 = Bundle By Name(cluster=w256, "Probe"=w254) -> (w255:T4)
                  }
                  frame True {
                    n156 = Bundle By Name(cluster=w259, "Probe"=0) -> (w258:T4)
                    n157 = call <vilib>:"Application Directory.vi"() -> ("Application Directory"=w266:path)
                    n158 = Path To String(path=w266) -> (string=w265:string)
                    n159 = Concatenate Strings(w265, "\\alarms_events\\") -> (w263:string)
                    n160 = String To Path(string=w263) -> (path=w262:path)
                    n161 = Build Path(base path=w262, name or relative path="Alarms.txt") -> (appended path=w261:path)
                    n162 = Open/Create/Replace File(file path (use dialog)=w261, operation (0:open)=T5."open or create", access (0:read/write)=enum16{"read/write", "read-only", "write-only"}."write-only") -> (refnum out=w284:refnum<file>, error out=w285:errorcluster)  [unwired: 3 in, 1 out]
                    n163 = Get Date/Time String() -> (date string=w273:string, time string=w271:string)  [unwired: 3 in]
                    n164 = Set File Position(refnum=w284, from (0:start)=enum16{"start", "end", "current"}."end", error in=w285) -> (refnum out=w281:refnum<file>, error out=w280:errorcluster)  [unwired: 1 in]
                    n165 = Format Into String(format string="%s %s %s %s %s %s %s %s", "CLIENT" ("format string"), "Date:" ("format string"), w273, "Time:" ("format string"), w271, "ALARM: " ("format string"), "Proba wlomania sie do systemu(3 razy zle haslo)" ("format string"), "\r\n") -> (resulting string=w268:string)  [unwired: 2 in, 1 out]
                    n166 = Write to Text File(file (use dialog)=w281, text=w268, error in=w280) -> (refnum out=w282:refnum<file>, error out=w283:errorcluster)  [unwired: 1 in, 1 out]
                    n167 = Close File(refnum=w282, error in=w283) -> ()  [unwired: 2 out]
                  }
                }
                n168 = Equal?(x=w252, y="") -> (x = y?=w248:bool)
                n169 = Equal?(x=w249, y="") -> (x = y?=w247:bool)
                n170 = Or(x=w248, y=w247) -> (x .or. y?=w246:bool)
                n171 = case shown="False" w246 {
                  frame False {
                    n172 = call "Display Message to User3"() -> ()  [unwired: 10 in, 2 out]
                  }
                  frame True {
                    n173 = call "Display Message to User4"() -> ()  [unwired: 10 in, 2 out]
                  }
                }
              }
              frame True {
                w287 = Tab_typeDef_user."Start_page" ("tab_control_user")
                n174 = Bundle By Name(cluster=w289, "tab_control_user"=w287) -> (w288:T4)
                n175 = local write "Tab Control"(w287) -> ()
                n176 = call "Display Message to User10"() -> ()  [unwired: 10 in, 2 out]
                "String" <- w286
              }
            }
          }
          event "register_btn": Value Change {
            w298 = "" ("first_name_rgstr")
            w307 = Tab_typeDef_user."Registration" ("tab_control_user")
            n177 = event-data() -> ()  [unwired: 1 in, 6 out]
            n178 = Bundle By Name(cluster=w308, "tab_control_user"=w307) -> (w306:T4)
            n179 = property on="first_name_rgstr" class="Str"(error in=w300, "Value"=w298) -> (error out=w304:errorcluster)  [unwired: 1 in, 1 out]
            n180 = local write "Tab Control"(w307) -> ()
            n181 = property on="last_name_rgstr" class="Str"(error in=w304, "Value"=w298) -> (error out=w303:errorcluster)  [unwired: 1 in, 1 out]
            n182 = property on="email_address_rgstr" class="Str"(error in=w303, "Value"=w298) -> (error out=w305:errorcluster)  [unwired: 1 in, 1 out]
            n183 = property on="username_rgstr" class="Str"(error in=w305, "Value"=w298) -> (error out=w302:errorcluster)  [unwired: 1 in, 1 out]
            n184 = property on="password_rgstr" class="Str"(error in=w302, "Value"=w298) -> (error out=w301:errorcluster)  [unwired: 1 in, 1 out]
            n185 = property on="rgstr_status" class="Str"(error in=w301, "Value"=w298) -> (error out=w299:errorcluster)  [unwired: 1 in, 1 out]
          }
          event "register_btn_rgstr": Value Change {
            n186 = event-data() -> ()  [unwired: 1 in, 6 out]
            n187 = call <vilib>:"Application Directory.vi"() -> ("Application Directory"=w319:path)
            n188 = Path To String(path=w319) -> (string=w318:string)
            n189 = Concatenate Strings(w318, "\\databases\\") -> (w316:string)
            n190 = flat-sequence {
              tunnel: "last_name_rgstr" -> [w328]
              tunnel: "first_name_rgstr" -> [w327]
              tunnel: [w330] -> w323
              tunnel: w309 -> [w329]
              tunnel: [w325] -> w322
              tunnel: w323 -> [w346]
              tunnel: [w345] -> w321
              tunnel: "password_rgstr" -> [w351]
              tunnel: [w342] -> _
              tunnel: "email_address_rgstr" -> [w350]
              tunnel: "last_name_rgstr" -> [w349]
              tunnel: "first_name_rgstr" -> [w348]
              tunnel: w322 -> [w344]
              tunnel: w309 -> [w343]
              tunnel: "username_rgstr" -> [w342]
              tunnel: w321 -> [w370]
              tunnel: w309 -> [w376]
              tunnel: "first_name_rgstr" -> [w375]
              tunnel: "last_name_rgstr" -> [w374]
              tunnel: "email_address_rgstr" -> [w373]
              tunnel: "username_rgstr" -> [w372]
              tunnel: "password_rgstr" -> [w371]
              frame #0 {
                n191 = call-poly <vilib>:"Read Delimited Spreadsheet.vi"("file path (dialog if empty)"=w329, "delimiter (\\t)"="," ("delimiter (\\t)")) -> ("all rows"=w331:string[][])  [unwired: 8 in, 5 out]
                n192 = for {
                  N -> [w333]
                  tunnel: w331 -> [w335] mode=indexing
                  tunnel: w328 -> [w339]
                  tunnel: w327 -> [w338]
                  tunnel: [w334] -> w330
                  tunnel: [w333] -> w324
                  stop <- w334 stop-if-true
                  n193 = Index Array(array=w335) -> (element #1=w341:string, element #2=w340:string)  [unwired: 2 in]
                  n194 = Equal?(x=w341, y=w339) -> (x = y?=w337:bool)
                  n195 = Equal?(x=w340, y=w338) -> (x = y?=w336:bool)
                  n196 = And(x=w337, y=w336) -> (x .and. y?=w334:bool)
                  n197 = case shown="True" w334 {
                    frame False {
                    }
                    frame True {
                      n198 = call "Display Message to User6"() -> ()  [unwired: 10 in, 2 out]
                    }
                  }
                }
                n199 = Equal?(x=w324, y=0) -> (x = y?=w325:bool)
              }
              frame #1 {
                w352 = "" ("delimiter (\\t)")
                n200 = case shown="True" w344 {
                  tunnel: w343 -> [_ w361]
                  frame False {
                  }
                  frame True {
                    n201 = Build Array("First Name", "Last Name", "Email", "Username", "Password") -> (w366:string[])
                    n202 = call-poly <vilib>:"Write Delimited Spreadsheet.vi"("file path (dialog if empty)"=w361, "1D data"=w366, "append to file? (new file:F)"=TRUE, "delimiter (\\t)"="," ("delimiter (\\t)")) -> ()  [unwired: 10 in, 2 out]
                  }
                }
                n203 = Equal?(x=w351, y=w352) -> (x = y?=w360:bool)
                n204 = Equal?(x=w342, y=w352) -> (x = y?=w359:bool)
                n205 = Equal?(x=w350, y=w352) -> (x = y?=w358:bool)
                n206 = Equal?(x=w349, y=w352) -> (x = y?=w357:bool)
                n207 = Equal?(x=w348, y=w352) -> (x = y?=w353:bool)
                n208 = Or(x=w360, y=w359) -> (x .or. y?=w356:bool)
                n209 = Or(x=w358, y=w357) -> (x .or. y?=w355:bool)
                n210 = Or(x=w356, y=w355) -> (x .or. y?=w354:bool)
                n211 = Or(x=w354, y=w353) -> (x .or. y?=w347:bool)
                n212 = case shown="True" w347 {
                  frame False {
                  }
                  frame True {
                    n213 = call "Display Message to User7"() -> ()  [unwired: 10 in, 2 out]
                  }
                }
                n214 = Or(x=w347, y=w346) -> (x .or. y?=w345:bool)
              }
              frame #2 {
                n215 = case shown="False" w370 {
                  tunnel: w376 -> [_ w383]
                  tunnel: w375 -> [_ w382]
                  tunnel: w374 -> [_ w381]
                  tunnel: w373 -> [_ w380]
                  tunnel: w372 -> [_ w379]
                  tunnel: w371 -> [_ w378]
                  frame True {
                  }
                  frame False {
                    n216 = Build Array(w382, w381, w380, w379, w378) -> (w386:string[])
                    n217 = call-poly <vilib>:"Write Delimited Spreadsheet.vi"("file path (dialog if empty)"=w383, "1D data"=w386, "append to file? (new file:F)"=TRUE, "delimiter (\\t)"="," ("delimiter (\\t)")) -> ()  [unwired: 10 in, 2 out]
                    "rgstr_status" <- "Registration was successful" ("rgstr_status")
                  }
                }
              }
            }
            n218 = String To Path(string=w316) -> (path=w315:path)
            n219 = Build Path(base path=w315, name or relative path="Clients_database.csv") -> (appended path=w309:path)
          }
          event "back_to_login_btn": Value Change {
            w387 = "" ("username_login")
            w392 = Tab_typeDef_user."Start_page" ("tab_control_user")
            n220 = event-data() -> ()  [unwired: 1 in, 6 out]
            n221 = property on="username_login" class="Str"(error in=w390, "Value"=w387) -> (error out=w389:errorcluster)  [unwired: 1 in, 1 out]
            n222 = property on="password_login" class="Str"(error in=w389, "Value"=w387) -> (error out=w388:errorcluster)  [unwired: 1 in, 1 out]
            n223 = Bundle By Name(cluster=w393, "tab_control_user"=w392) -> (w391:T4)
            n224 = local write "Tab Control"(w392) -> ()
          }
        }
      }
      frame "PROCESS" {
      }
      frame "EXIT" {
      }
    }
    n225 = Unbundle By Name(w11) -> ("status"=w13:bool)
    n226 = Or(x=w13, y=w12) -> (x .or. y?=w10:bool)
  }
  n227 = flat-sequence {
    tunnel: w2 -> [w402]
    frame #0 {
      n228 = call <vilib>:"Simple Error Handler.vi"("error in (no error)"=w402) -> ()  [unwired: 4 in, 5 out]
    }
  }
